vi "setSummaryState.vi"(10 "SummaryStates":T1, 11 "Model in":refnum<class "Model.lvclass">) -> (3 "Model out":refnum<class "Model.lvclass">)   [LabVIEW 2016, in "Model.lvclass"]
uses:
  Model.lvclass
  DataTypes/Topics/Parts/SummaryStates.ctl
  Model.lvclass/Model.ctl
  DataTypes/Topics/M1M3SupportTopics.lvlib
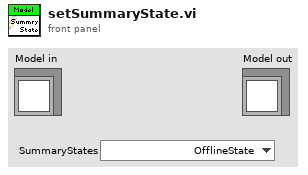
[diagram p1: front panel]
types:
  T1 = typedef "M1M3SupportTopics.lvlib/SummaryStates.ctl" = enum16{"OfflineState", "StandbyState", "DisabledState", "EnabledState", "FaultState"}
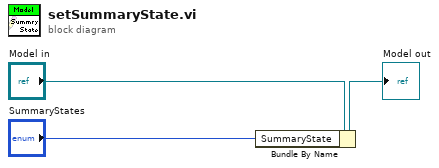
[diagram p0: block diagram]
diagram:
  n1 = Bundle By Name(cluster="Model in", "SummaryState"="SummaryStates") -> (→"Model out":refnum<class "Model.lvclass">)
